vi "E2-1.vi"() -> ()   [LabVIEW 2011]
panel:
  out "나중 속도":dbl
  in  "힘이 가해진 시간":dbl
  in  "질량":dbl
  in  "힘":dbl
  in  "초기 속도":dbl
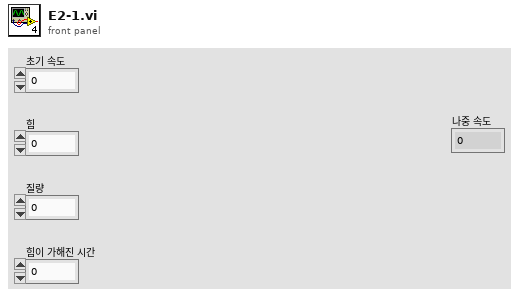
[diagram p1: front panel]
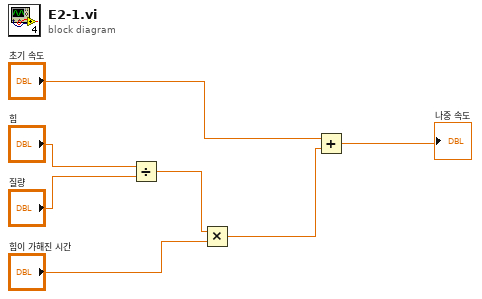
[diagram p0: block diagram]
diagram:
  n1 = Divide(x="힘", y="질량") -> (x/y=w5:dbl)
  n2 = Multiply(x=w5, y="힘이 가해진 시간") -> (x*y=w3:dbl)
  n3 = Add(x="초기 속도", y=w3) -> (x+y=→"나중 속도":dbl)
